vi "Report Shake Data.vi"(8 "error in (no error)":errorcluster, 9 "Amplitude (g)":dbl, 10 "Frequency (Hz)":dbl, 11 "Executive in":refnum<class "Executive.lvclass">) -> (0 "error out":errorcluster, 3 "Executive out":refnum<class "Executive.lvclass">)   [LabVIEW 2020, in "Executive.lvlib" / "Executive.lvclass"]
uses:
  Executive.lvclass
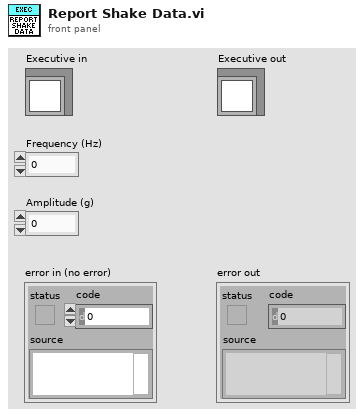
[diagram p1: front panel]
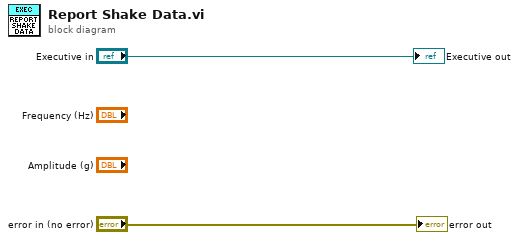
[diagram p0: block diagram]
diagram:
  "error out" <- "error in (no error)"
  "Executive out" <- "Executive in"
